vi "Convert Available to Used.vi"(5 "Size":u32, 8 "Minimum Amount Available":u32, 9 "Current Amount Available":u32) -> (2 "Maximum Amount Used":u32, 3 "Current Amount Used":u32)   [LabVIEW 2016]
doc: "This SubVI converts the reported amount of available elements in the FPGA FIFO to the amount of elements of the FIFO being Used."
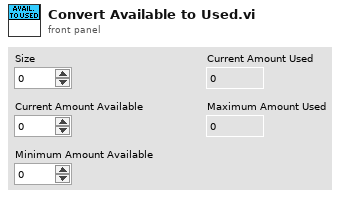
[diagram p1: front panel]
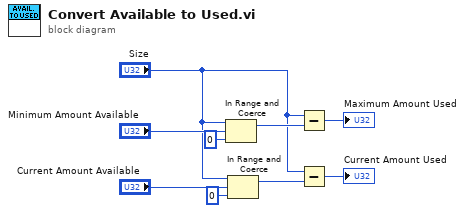
[diagram p0: block diagram]
diagram:
  n1 = In Range and Coerce(upper limit="Size", x="Minimum Amount Available", lower limit=u32 0) -> (coerced(x)=w5:u32)  [unwired: 1 out]
  n2 = In Range and Coerce(upper limit="Size", x="Current Amount Available", lower limit=u32 0) -> (coerced(x)=w4:u32)  [unwired: 1 out]
  n3 = Subtract(x="Size", y=w5) -> (x-y=→"Maximum Amount Used":u32)
  n4 = Subtract(x="Size", y=w4) -> (x-y=→"Current Amount Used":u32)
